vi "Parse 19-1.vi"(11 "String":string) -> (3 "Scanners":T1[](array[typedef]))   [LabVIEW 2020]
uses:
  Scanner.ctl
  Vec3.ctl
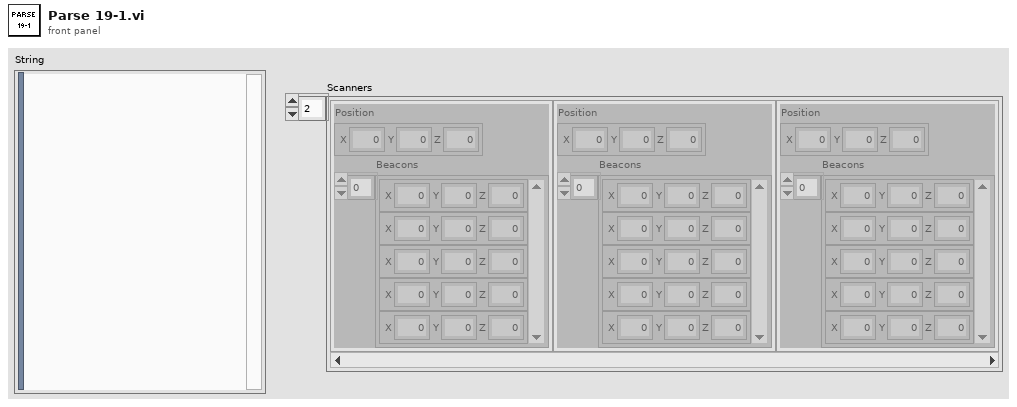
[diagram p1: front panel]
types:
  T1 = typedef "Scanner.ctl" = cluster{"Position":T2, "Beacons":T2[]}
  T2 = typedef "Vec3.ctl" = cluster{"X":dbl, "Y":dbl, "Z":dbl}
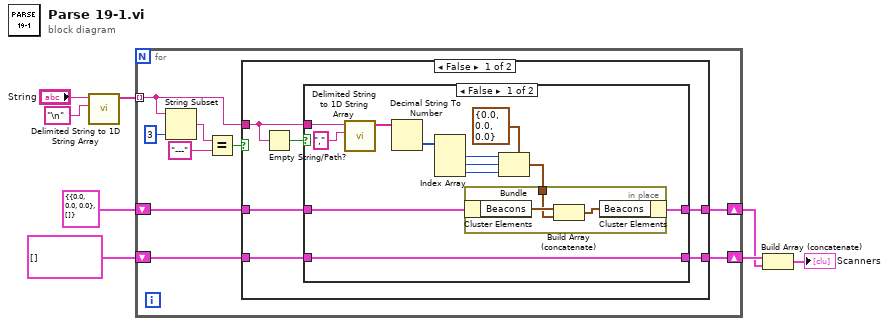
[diagram p0: block diagram]
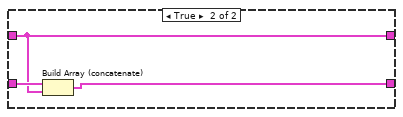
[diagram p2: hidden frame]
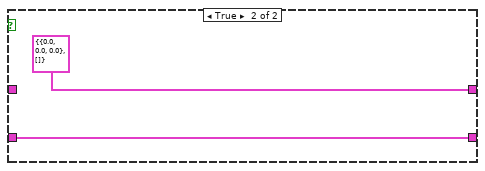
[diagram p3: hidden frame]
diagram:
  n1 = call <vilib>:"Delimited String to 1D String Array.vi"("delimiter"="\n", "delimited string"="String") -> ("string array"=w6:string[])  [unwired: 9 in]
  n2 = for {
    tunnel: w6 -> [w9] mode=indexing
    shift-right: [w11] -> w4
    shift-left: T1[] [] -> [w12]
    shift-right: [w13] -> w1
    shift-left: T1 {"Position"={"X"=0.0, "Y"=0.0, "Z"=0.0}, "Beacons"=[]} ("Scanner") -> [w14]
    n3 = String Subset(string=w9, length (rest)=3 ("length (rest)")) -> (substring=w10:string)  [unwired: 1 in]
    n4 = Equal?(x=w10, y="---") -> (x = y?=w15:bool)
    n5 = case shown="False" w15 {
      tunnel: w14 -> [w22 _]
      tunnel: [w19 T1 {"Position"={"X"=0.0, "Y"=0.0, "Z"=0.0}, "Beacons"=[]} ("Scanner")] -> w13
      tunnel: w12 -> [w21 w42]
      tunnel: [w20 w42] -> w11
      tunnel: w9 -> [w18 _]
      frame False {
        n6 = Empty String/Path?(string/path=w18) -> (empty?=w23:bool)
        n7 = case shown="False" w23 {
          tunnel: w22 -> [w26 w39]
          tunnel: w21 -> [w31 w41]
          tunnel: [w31 w40] -> w20
          tunnel: [w24 w39] -> w19
          tunnel: w18 -> [w35 _]
          frame False {
            n8 = call <vilib>:"Delimited String to 1D String Array.vi"("delimiter"=",", "delimited string"=w35) -> ("string array"=w33:string[])  [unwired: 9 in]
            n9 = Decimal String To Number(string=w33) -> (number=w32:i32[])  [unwired: 2 in, 1 out]
            n10 = Index Array(array=w32) -> (element #1=w29:i32, element #2=w28:i32, element #3=w27:i32)  [unwired: 3 in]
            n11 = Bundle(cluster=T2 {"X"=0.0, "Y"=0.0, "Z"=0.0} ("Position"), "X"=w29, "Y"=w28, "Z"=w27) -> (w25:T2)
            n12 = in-place {
              in-place-border: w25 -> [w37]
              n13 = in-place-cluster #1(w26) -> ("Beacons"=w38:T2[])
              n14 = Build Array (concatenate)(w38, w37) -> (w36:T2[])
              n15 = in-place-cluster #1("Beacons"=w36) -> (w24:T1)
            }
          }
          frame True {
            n16 = Build Array (concatenate)(w41, w39) -> (w40:T1[])
          }
        }
      }
      frame True {
      }
    }
  }
  n17 = Build Array (concatenate)(w4, w1) -> (→"Scanners":T1[])
